vi "Write VSSParams.vi"(8 "error in (no error)":errorcluster, 10 "VSSParams":T1={"Robots ids"={"Goalie"=enum."0", "Attacker"=enum."1", "Defender"=enum."2"}}, 11 "Parameters in":refnum<class "Parameters.lvclass">) -> (0 "error out":errorcluster, 3 "Parameters out":refnum<class "Parameters.lvclass">)   [LabVIEW 2023, in "Parameters.lvclass"]
uses:
  Parameters.lvclass
  Parameters.lvclass/Parameters.ctl
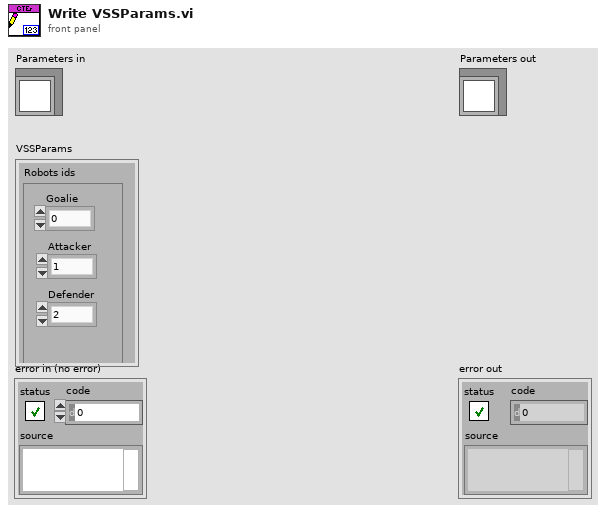
[diagram p1: front panel]
types:
  T1 = cluster{"Robots ids":cluster{"Goalie":enum16{"auto", "5", "4", "3", "2", "1", "0"}, "Attacker":enum16{"auto", "5", "4", "3", "2", "1", "0"}, "Defender":enum16{"auto", "5", "4", "3", "2", "1", "0"}}}
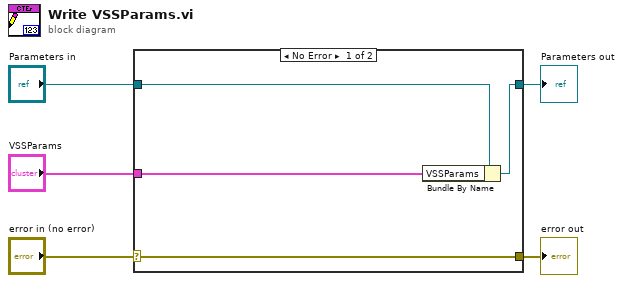
[diagram p0: block diagram]
diagram:
  n1 = case shown="No Error" "error in (no error)" {
    selector: "error in (no error)" -> [w9 w10]
    tunnel: [w9 w10] -> w4
    tunnel: [w7 w11] -> w2
    tunnel: "Parameters in" -> [w8 w11]
    tunnel: "VSSParams" -> [w6 _]
    frame No Error {
      n2 = Bundle By Name(cluster=w8, "VSSParams"=w6) -> (w7:refnum<class "Parameters.lvclass">)
    }
    frame Error {
    }
  }
  "error out" <- w4
  "Parameters out" <- w2
